vi "SSC DCPower Get SMU Models.vi"(0 "DCPower SSC in":T1[](array[typedef]), 11 "error in":errorcluster) -> (4 "DCPower SSC out":T1[](array[typedef]), 6 "SMU Models":string[](array[string]), 15 "error out":errorcluster)   [LabVIEW 2020]
doc: "This VI gets the 4-digit numerical model number for each DCPower Session.\n\nFor example, this will return \"4139\" for a PXIe-4139 SMU."
uses:
  SSC DCPower.ctl
  <vilib>/regexp/Match Regular Expression.xnode
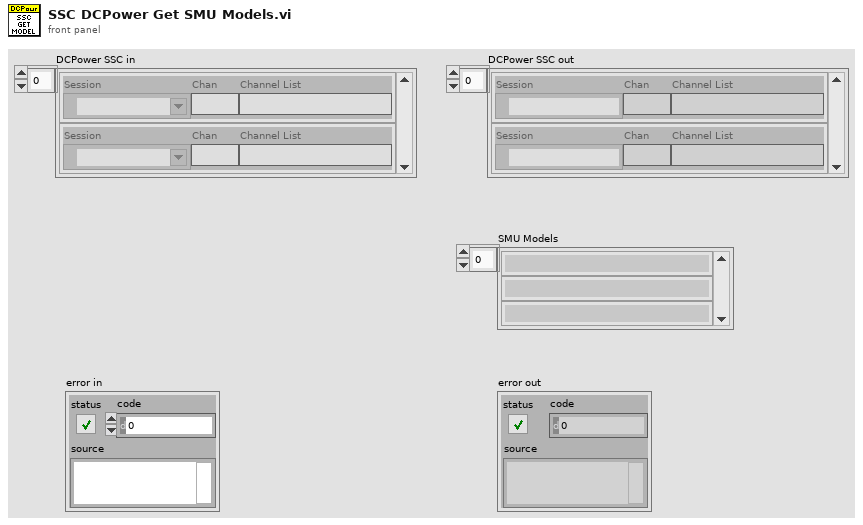
[diagram p1: front panel]
types:
  T1 = typedef "SSC DCPower.ctl" = cluster{"Session":refnum<k15>, "Chan":string, "Channel List":string}
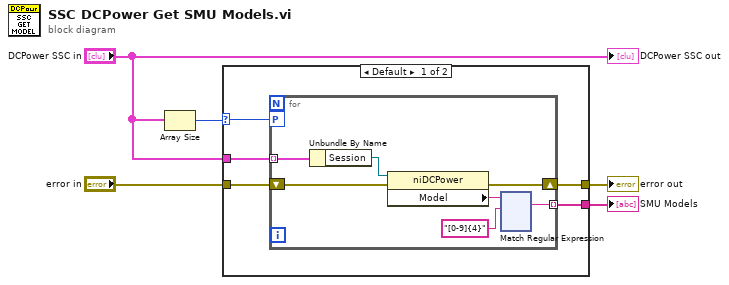
[diagram p0: block diagram]
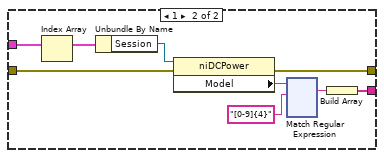
[diagram p2: hidden frame]
diagram:
  n1 = Array Size(array="DCPower SSC in") -> (size(s)=w1:i32)
  n2 = case shown="Default" w1 {
    selector: w1 -> [w6 _]
    tunnel: "DCPower SSC in" -> [w10 w140]
    tunnel: "error in" -> [w9 w139]
    tunnel: [w8 w138] -> w4
    tunnel: [w7 w133] -> w3
    frame Default {
      n3 = for {
        tunnel: w10 -> [w17] mode=indexing
        shift-right: [w14] -> w8
        shift-left: w9 -> [w15]
        tunnel: [w11] -> w7 mode=indexing
        workers-P: w6 -> [_]
        n4 = Unbundle By Name(w17) -> ("Session"=w16:refnum<k15>)
        n5 = property class="niDCPower"(reference=w16, error in=w15) -> (error out=w14:errorcluster, "Model"=w13:string)  [unwired: 1 out]
        n6 = xnode "Match Regular Expression"("input string"=w13, "regular expression"="[0-9]{4}") -> ("whole match"=w11:string)  [unwired: 4 in, 4 out]
      }
    }
    frame 1 {
      n7 = Index Array(array=w140) -> (element=w132:T1)  [unwired: 1 in]
      n8 = Unbundle By Name(w132) -> ("Session"=w136:refnum<k15>)
      n9 = property class="niDCPower"(reference=w136, error in=w139) -> (error out=w138:errorcluster, "Model"=w135:string)  [unwired: 1 out]
      n10 = xnode "Match Regular Expression"("input string"=w135, "regular expression"="[0-9]{4}") -> ("whole match"=w137:string)  [unwired: 4 in, 4 out]
      n11 = Build Array(w137) -> (w133:string[])
    }
  }
  "error out" <- w4
  "SMU Models" <- w3
  "DCPower SSC out" <- "DCPower SSC in"
